vi "Prepare LV to Use Icon Editor Source.vi"   [LabVIEW 2023]
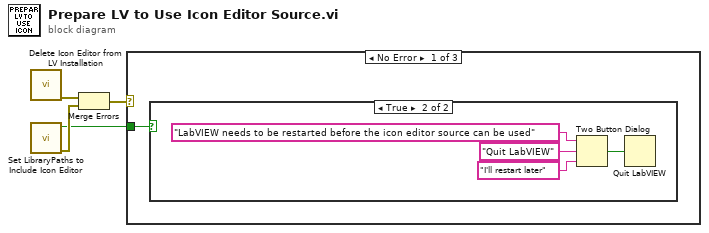
[diagram p0: block diagram]
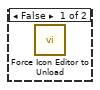
[diagram p2: hidden frame]
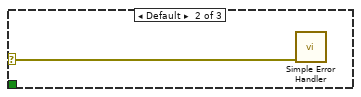
[diagram p3: hidden frame]
diagram:
  n1 = call "Delete Icon Editor from LV Installation.vi"() -> ("error out"=w4:errorcluster)  [unwired: 10 in, 1 out]
  n2 = call "Set LibraryPaths to Include Icon Editor.vi"() -> ("error out"=w2:errorcluster, "config modified?"=w1:bool)  [unwired: 10 in]
  n3 = Merge Errors(w4, w2) -> (w3:errorcluster)
  n4 = case shown="No Error" w3 {
    selector: w3 -> [_ w10 _]
    tunnel: w1 -> [w5 _ _]
    frame No Error {
      n5 = case shown="True" w5 {
        frame False {
          n6 = call "Force Icon Editor to Unload.vi"() -> ()  [unwired: 12 in]
        }
        frame True {
          n7 = Two Button Dialog(message="LabVIEW needs to be restarted before the icon editor source can be used", 1:"I'll restart later" ("F button name (\"Cancel\")"), 2:"Quit LabVIEW" ("T button name (\"OK\")")) -> (T button?=w9:bool)
          n8 = Quit LabVIEW(quit? (T)=w9) -> ()
        }
      }
    }
    frame Default {
      n9 = call <vilib>:"Simple Error Handler.vi"("error in (no error)"=w10) -> ()  [unwired: 4 in, 5 out]
    }
    frame Error {
      # "User cancelled, no further interaction needed"
    }
  }
